vi "get VISA RSC.vi"(8 "error in (no error)":errorcluster caption="错误输入（无错误）", 11 "DGUS 输入":refnum<class "DGUS.lvclass">) -> (0 "error out":errorcluster caption="错误输出", 2 "VISA资源名称":refnum<visa-resource-name>, 3 "DGUS 输出":refnum<class "DGUS.lvclass">)   [LabVIEW 2016, in "DGUS.lvlib" / "DGUS.lvclass"]
uses:
  DGUS.lvclass
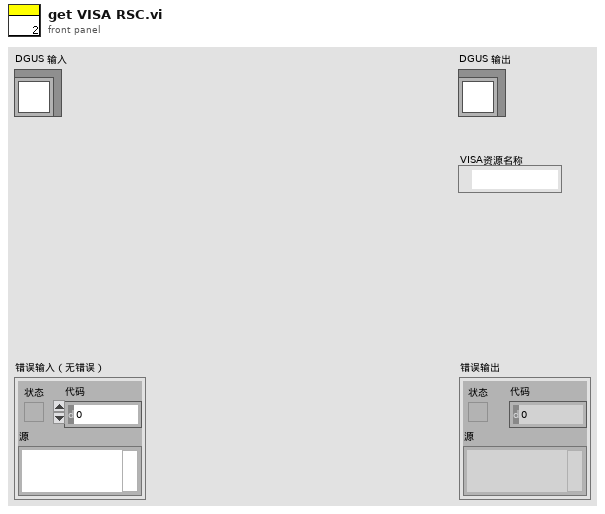
[diagram p1: front panel]
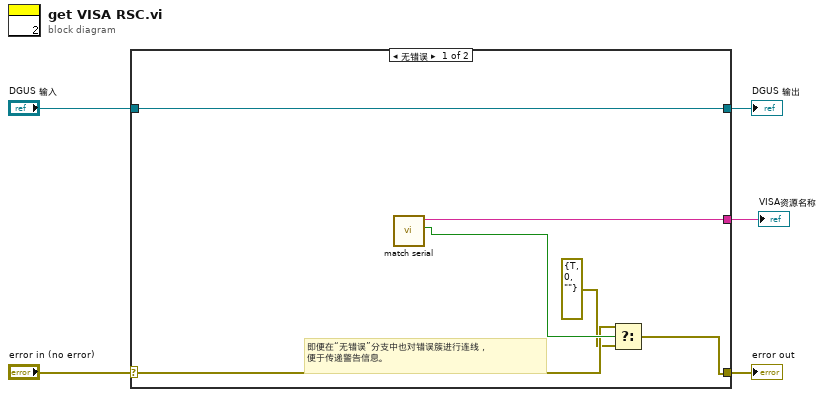
[diagram p0: block diagram]
diagram:
  n1 = case shown="无错误" "error in (no error)" {
    selector: "error in (no error)" -> [w8 w13]
    tunnel: [w6 w13] -> w4
    tunnel: [w11 w12] -> w2
    tunnel: "DGUS 输入" -> [w11 w12]
    tunnel: [w10 _] -> w1
    frame No Error {
      # "即便在“无错误”分支中也对错误簇进行连线，\n便于传递警告信息。"
      n2 = call "match serial.vi"() -> ("match?"=w9:bool, "配置串口"=w10:string)  [unwired: 10 in]
      n3 = Select(t=w8, s=w9, f=errorcluster {"status"=TRUE, "code"=0, "source"=""}) -> (s? t:f=w6:errorcluster)
    }
    frame Error {
    }
  }
  "error out" <- w4
  "DGUS 输出" <- w2
  "VISA资源名称" <- w1
